vi "Load Scaffold Config.vi"(8 "error in (no error)":errorcluster, 11 "Path":path) -> (0 "error out":errorcluster, 3 "Folders":T1[](array[typedef]))   [LabVIEW 2020, in "Negentropic IDE.lvlib"]
uses:
  Negentropic IDE.lvlib
  Folder Config.ctl
  Scope.ctl
  <vilib>/Utility/config.llb/Read Key (String).vi
  <vilib>/Utility/config.llb/NI_LVConfig.lvlib
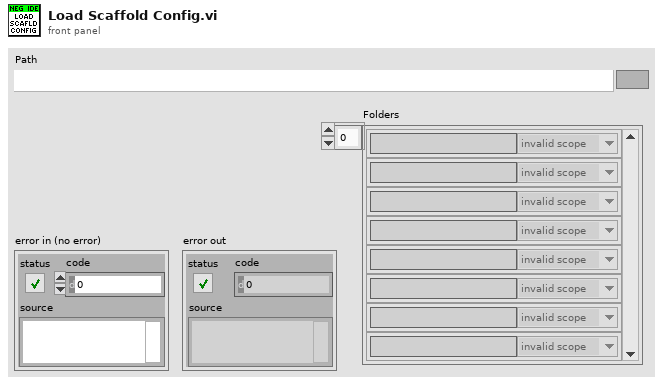
[diagram p1: front panel]
types:
  T1 = typedef "Negentropic IDE.lvlib/Folder Config.ctl" = cluster{"Path":string, "Scope":T2}
  T2 = typedef "Negentropic IDE.lvlib/Scope.ctl" = enum32{"invalid scope", "public", "private", "protected", "community"}
  T3 = typedef "NI_LVConfig.lvlib/Config Data RefNum.ctl" = refnum<k1>
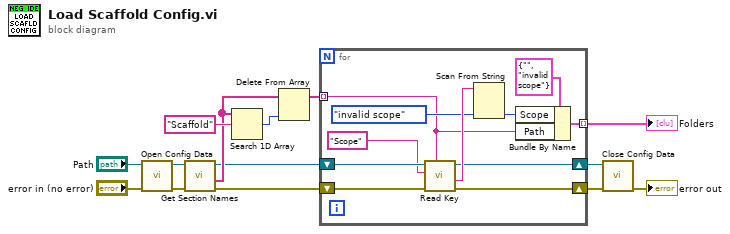
[diagram p0: block diagram]
diagram:
  n1 = call <vilib>:"Open Config Data.vi"("error in (no error)"="error in (no error)", "configuration file path"="Path") -> ("error out"=w12:errorcluster, "refnum"=w11:T3)  [unwired: 7 in, 1 out]
  n2 = call <vilib>:"Get Section Names.vi"("error in (no error)"=w12, "refnum"=w11) -> ("error out"=w6:errorcluster, "section names"=w9:string[], "refnum out"=w7:T3)  [unwired: 7 in]
  n3 = Search 1D Array(1D array=w9, element="Scaffold") -> (index of element=w8:i32)  [unwired: 1 in]
  n4 = Delete From Array(array=w9, index=w8) -> (array with subset deleted=w5:string[])  [unwired: 1 in, 1 out]
  n5 = for {
    shift-right: [w16] -> w3
    shift-left: w7 -> [w24]
    shift-right: [w15] -> w2
    shift-left: w6 -> [w25]
    tunnel: w5 -> [w18] mode=indexing
    tunnel: [w17] -> w4 mode=indexing
    n6 = call-poly <vilib>:"Read Key.vi"("section"=w18, "error in (no error)"=w25, "key"="Scope", "refnum"=w24) -> ("error out"=w15:errorcluster, "value"=w22:string, "refnum out"=w16:T3)  [unwired: 4 in, 1 out]
    n7 = Scan From String(input string=w22, default 1=Scope."invalid scope" ("Scope")) -> (output 1=w19:T2)  [unwired: 3 in, 3 out]
    n8 = Bundle By Name(cluster=T1 {"Path"="", "Scope"=enum."invalid scope"} ("Folder Config"), "Scope"=w19, "Path"=w18) -> (w17:T1)
  }
  "Folders" <- w4
  n9 = call <vilib>:"Close Config Data.vi"("error in (no error)"=w2, "refnum"=w3) -> ("error out"=→"error out":errorcluster)  [unwired: 8 in, 1 out]
